vi "OSU_Sample.vi"() -> ()   [LabVIEW 2017]
uses:
  D:/test/FULLband-sts/Fullband_Sample/DLL/InstrumentDLL.dll
  DLL/InstrumentDLL.dll
panel:
  out "OSU":refnum<k24>
  in  "btn_Switch":bool
  in  "channel":u16(ring) items=["", "Ch1", "Ch2", "Ch3", "Ch4"]
  in  "OSU Control device name":u16(ring)
  in  "Btn_DisConnect":bool
  in  "Btn_Connect":bool
  # "1. Connect"
  # "2. Setting function"
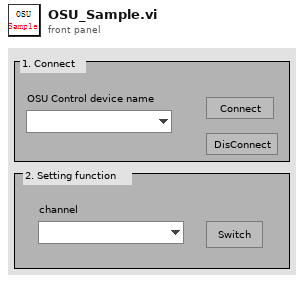
[diagram p1: front panel]
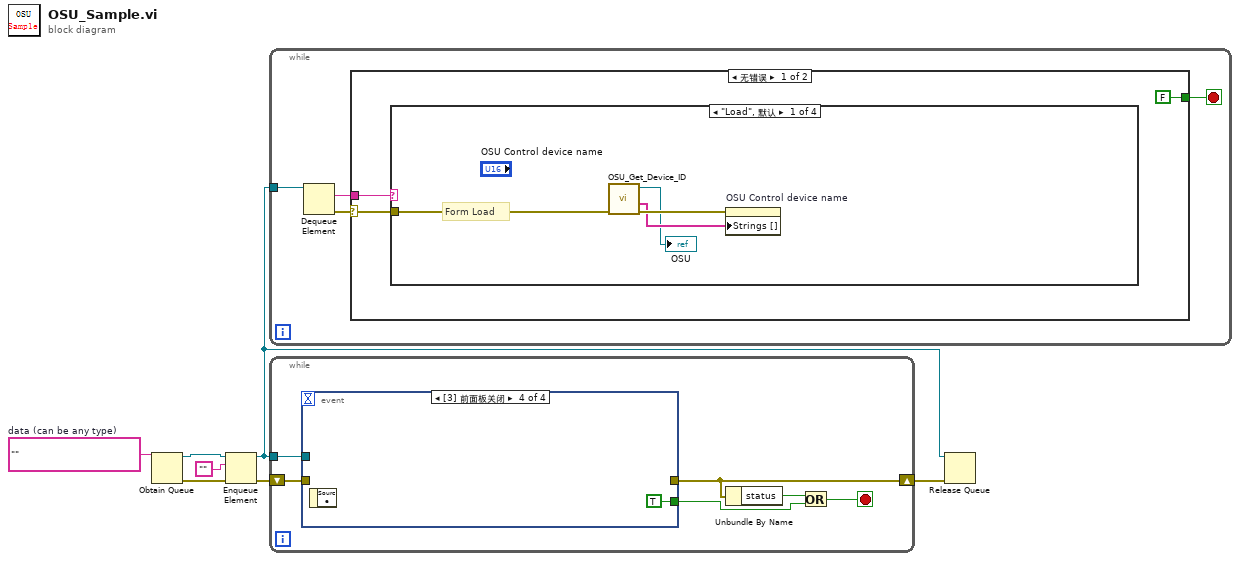
[diagram p0: block diagram]
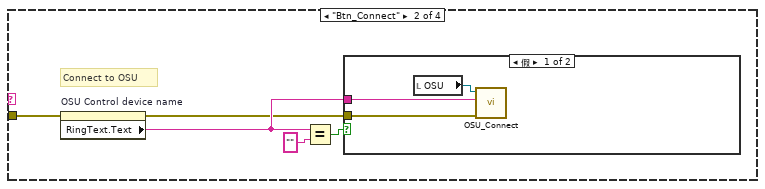
[diagram p2: hidden frame]
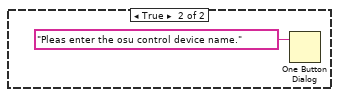
[diagram p3: hidden frame]
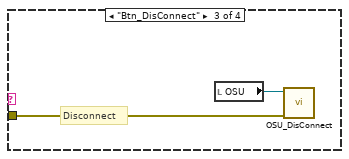
[diagram p4: hidden frame]
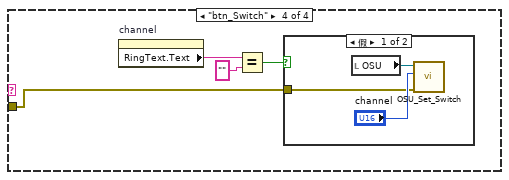
[diagram p5: hidden frame]
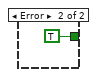
[diagram p7: hidden frame]
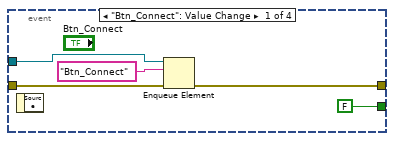
[diagram p8: hidden frame]
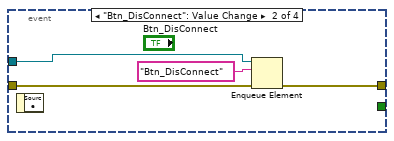
[diagram p9: hidden frame]
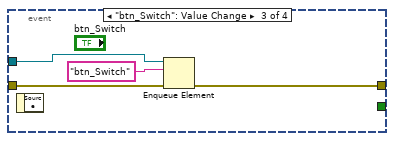
[diagram p10: hidden frame]
diagram:
  w6 = ""  # data (can be any type)
  n1 = Obtain Queue(element data type=w6) -> (queue out=w5:refnum<queue>, error out=w7:errorcluster)  [unwired: 4 in, 1 out]
  n2 = Enqueue Element(queue=w5, element="", error in (no error)=w7) -> (queue out=w1:refnum<queue>, error out=w3:errorcluster)  [unwired: 1 in, 1 out]
  n3 = while {
    tunnel: w1 -> [w11]
    stop <- w8 stop-if-true
    n4 = Dequeue Element(queue=w11) -> (element=w9:string, error out=w10:errorcluster)  [unwired: 2 in, 2 out]
    n5 = case shown="无错误" w10 {
      selector: w10 -> [w12 _]
      tunnel: w9 -> [w14 _]
      tunnel: [FALSE TRUE] -> w8
      frame No Error {
        n6 = case shown="\"Load\", 默认" w14 {
          tunnel: w12 -> [w18 w23 w28 w30]
          frame "Load", Default {
            # "Form Load"
            n7 = call "OSU_Get_Device_ID.vi"("error in (no error)"=w18) -> ("error out"=w17:errorcluster, "id"=w16:string[], "Reference out"=→"OSU":refnum<k24>)  [unwired: 8 in]
            n8 = property on="OSU Control device name" class="Ring (严格)"(error in=w17, "Strings []"=w16) -> ()  [unwired: 1 in, 2 out]
          }
          frame "Btn_Connect" {
            # "Connect to OSU"
            n9 = property on="OSU Control device name" class="Ring (严格)"(error in=w23) -> (error out=w19:errorcluster, "RingText.Text"=w20:string)  [unwired: 1 in, 1 out]
            n10 = Equal?(x=w20, y="") -> (x = y?=w21:bool)
            n11 = case shown="假" w21 {
              tunnel: w20 -> [w25 _]
              tunnel: w19 -> [w24 _]
              frame False {
                n12 = local read "OSU"() -> (w26:refnum<k24>)
                n13 = call "OSU_Connect.vi"("error in (no error)"=w24, "DeviceName"=w25, ".NET Reference in"=w26) -> ()  [unwired: 6 in, 3 out]
              }
              frame True {
                n14 = One Button Dialog(message="Pleas enter the osu control device name." ("消息")) -> ()  [unwired: 1 in, 1 out]
              }
            }
          }
          frame "Btn_DisConnect" {
            # "Disconnect"
            n15 = local read "OSU"() -> (w29:refnum<k24>)
            n16 = call "OSU_DisConnect.vi"("error in (no error)"=w28, ".NET Reference in"=w29) -> ()  [unwired: 8 in, 2 out]
          }
          frame "btn_Switch" {
            n17 = property on="channel" class="Ring (严格)"() -> ("RingText.Text"=w33:string)  [unwired: 2 in, 2 out]
            n18 = Equal?(x=w33, y="") -> (x = y?=w31:bool)
            n19 = case shown="假" w31 {
              tunnel: w30 -> [w34 _]
              frame False {
                n20 = local read "OSU"() -> (w36:refnum<k24>)
                n21 = call "OSU_Set_Switch.vi"("error in (no error)"=w34, "channel"="channel", ".NET Reference in"=w36) -> ()  [unwired: 7 in, 2 out]
              }
              frame True {
              }
            }
          }
        }
      }
      frame Error {
      }
    }
  }
  n22 = while {
    tunnel: w1 -> [w42]
    shift-right: [w40] -> w2
    shift-left: w3 -> [w41]
    stop <- w39 stop-if-true
    n23 = event shown="[3] 前面板关闭" {
      selector: _ -> [_ _ _ _]
      dyn-events: _ -> [_ _ _ _]
      timeout: _ -> [_ _ _ _]
      tunnel: w42 -> [w48 w51 w56 _]
      tunnel: w41 -> [w47 w50 w55 _]
      tunnel: [w46 w49 w54 _] -> w40
      tunnel: [FALSE ("y") _ _ TRUE ("y")] -> w38
      event "Btn_Connect": Value Change {
        n24 = event-data() -> ()  [unwired: 1 in, 1 out]
        n25 = Enqueue Element(queue=w48, element="Btn_Connect" ("元素"), error in (no error)=w47) -> (error out=w46:errorcluster)  [unwired: 1 in, 2 out]
      }
      event "Btn_DisConnect": Value Change {
        n26 = event-data() -> ()  [unwired: 1 in, 1 out]
        n27 = Enqueue Element(queue=w51, element="Btn_DisConnect" ("元素"), error in (no error)=w50) -> (error out=w49:errorcluster)  [unwired: 1 in, 2 out]
      }
      event "btn_Switch": Value Change {
        n28 = event-data() -> ()  [unwired: 1 in, 1 out]
        n29 = Enqueue Element(queue=w56, element="btn_Switch" ("元素"), error in (no error)=w55) -> (error out=w54:errorcluster)  [unwired: 1 in, 2 out]
      }
      event Panel Close {
        n30 = event-data() -> ()  [unwired: 1 in, 1 out]
      }
    }
    n31 = Unbundle By Name(w40) -> ("status"=w43:bool)
    n32 = Or(x=w43, y=w38) -> (x .or. y?=w39:bool)
  }
  n33 = Release Queue(queue=w1, error in (no error)=w2) -> ()  [unwired: 1 in, 3 out]
